vi "AutoGetAvailableRoutines.vi"(1 "AllAutoRoutines":T8, 2 "AutoStartingPosition":T7) -> (0 "AvailableRoutines":T1)   [LabVIEW 2017]
uses:
  TypeDef/AutoRoutines.ctl
  TypeDef/AutoRoutineSet.ctl
  TypeDef/AutoStep.ctl
  TypeDef/AutoWaypointType.ctl
  Pathfinder/Pathfinder-LabVIEW/Pathfinder-Lib/VIs/Waypoint.ctl
  Implements/Arm/TypeDefs/ArmTargetPosition.ctl
  Implements/TypeDefs/IntakeState.ctl
  TypeDef/AutoStartingPositions.ctl
  Pathfinder/Pathfinder-LabVIEW/Pathfinder-Lib/Pathfinder.lvlib
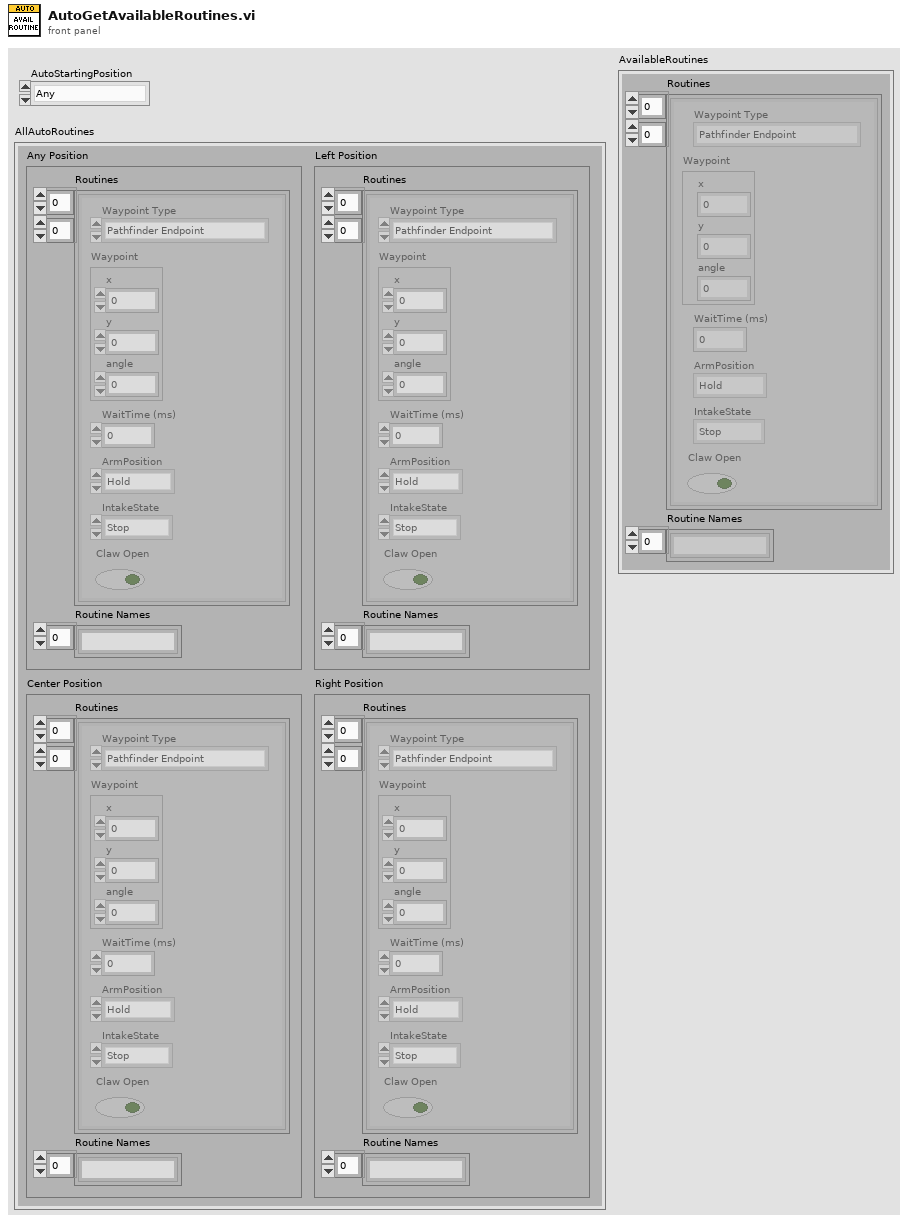
[diagram p1: front panel]
types:
  T1 = typedef "AutoRoutineSet.ctl" = cluster{"Routines":T2[][], "Routine Names":string[]}
  T2 = typedef "AutoStep.ctl" = cluster{"Waypoint Type":T3, "Waypoint":T4, "WaitTime (ms)":u16, "ArmPosition":T5, "IntakeState":T6, "Claw Open":bool}
  T3 = typedef "AutoWaypointType.ctl" = enum16{"Pathfinder Endpoint", "Pathfinder Waypoint", "Zero-Radius Turn Endpoint", "Stationary", "Vision Assist Endpoint", "Stop"}
  T4 = typedef "Pathfinder.lvlib/Waypoint.ctl" = cluster{"x":dbl, "y":dbl, "angle":dbl}
  T5 = typedef "ArmTargetPosition.ctl" = enum16{"Hold", "Switch", "Scale Low", "Scale High", "Climb", "Back Place"}
  T6 = typedef "IntakeState.ctl" = enum16{"Stop", "Forward", "Reverse", "Forward Open"}
  T7 = typedef "AutoStartingPositions.ctl" = enum16{"Any", "Left", "Center", "Right"}
  T8 = typedef "AutoRoutines.ctl" = cluster{"Any Position":T1, "Left Position":T1, "Center Position":T1, "Right Position":T1}
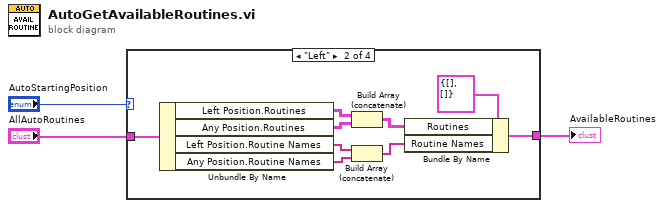
[diagram p0: block diagram]
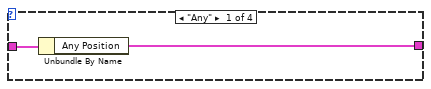
[diagram p2: hidden frame]
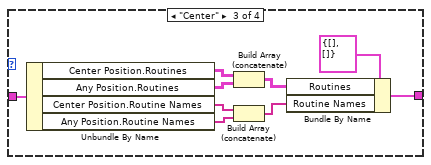
[diagram p3: hidden frame]
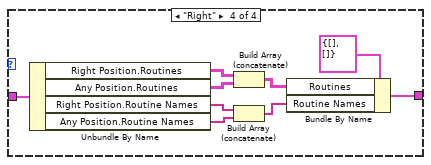
[diagram p4: hidden frame]
diagram:
  n1 = case shown="\"Left\"" "AutoStartingPosition" {
    tunnel: "AllAutoRoutines" -> [w5 w14 w23 w32]
    tunnel: [w4 w6 w15 w24] -> w1
    frame "Any" {
      n2 = Unbundle By Name(w5) -> ("Any Position"=w4:T1)
    }
    frame "Left" {
      n3 = Unbundle By Name(w14) -> ("Left Position.Routines"=w11:T2[][], "Any Position.Routines"=w10:T2[][], "Left Position.Routine Names"=w13:string[], "Any Position.Routine Names"=w12:string[])
      n4 = Build Array (concatenate)(w11, w10) -> (w8:T2[][])
      n5 = Build Array (concatenate)(w13, w12) -> (w7:string[])
      n6 = Bundle By Name(cluster=T1 {"Routines"=[], "Routine Names"=[]} ("Any Position"), "Routines"=w8, "Routine Names"=w7) -> (w6:T1)
    }
    frame "Center" {
      n7 = Unbundle By Name(w23) -> ("Center Position.Routines"=w20:T2[][], "Any Position.Routines"=w19:T2[][], "Center Position.Routine Names"=w22:string[], "Any Position.Routine Names"=w21:string[])
      n8 = Build Array (concatenate)(w20, w19) -> (w17:T2[][])
      n9 = Build Array (concatenate)(w22, w21) -> (w16:string[])
      n10 = Bundle By Name(cluster=T1 {"Routines"=[], "Routine Names"=[]} ("Any Position"), "Routines"=w17, "Routine Names"=w16) -> (w15:T1)
    }
    frame "Right" {
      n11 = Unbundle By Name(w32) -> ("Right Position.Routines"=w29:T2[][], "Any Position.Routines"=w28:T2[][], "Right Position.Routine Names"=w31:string[], "Any Position.Routine Names"=w30:string[])
      n12 = Build Array (concatenate)(w29, w28) -> (w26:T2[][])
      n13 = Build Array (concatenate)(w31, w30) -> (w25:string[])
      n14 = Bundle By Name(cluster=T1 {"Routines"=[], "Routine Names"=[]} ("Any Position"), "Routines"=w26, "Routine Names"=w25) -> (w24:T1)
    }
  }
  "AvailableRoutines" <- w1
